vi "Get Events.vi"(8 "error in (no error)":errorcluster, 11 "Series Actor in":refnum<class "Series Actor.lvclass">) -> (0 "error out":errorcluster, 2 "Events":cluster{"Stop":refnum<user-event>}, 3 "Series Actor out":refnum<class "Series Actor.lvclass">)   [LabVIEW 2023, in "Series Actor.lvlib" / "Series Actor.lvclass"]
uses:
  Series Actor.lvclass
  Series Actor.lvclass/Series Actor.ctl
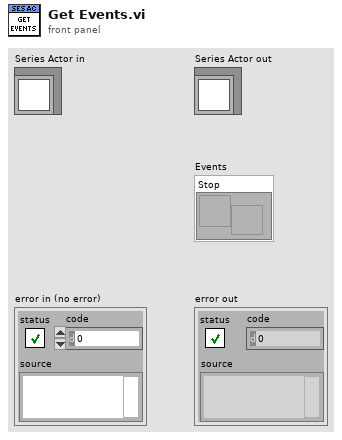
[diagram p1: front panel]
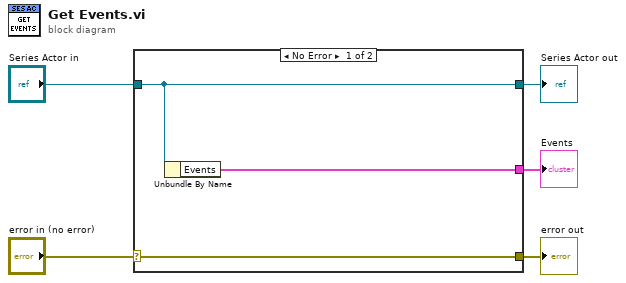
[diagram p0: block diagram]
diagram:
  n1 = case shown="No Error" "error in (no error)" {
    selector: "error in (no error)" -> [w8 w9]
    tunnel: [w8 w9] -> w4
    tunnel: [w7 w10] -> w2
    tunnel: "Series Actor in" -> [w7 w10]
    tunnel: [w6 _] -> w1
    frame No Error {
      n2 = Unbundle By Name(w7) -> ("Events"=w6:cluster{"Stop":refnum<user-event>})
    }
    frame Error {
    }
  }
  "error out" <- w4
  "Series Actor out" <- w2
  "Events" <- w1
